vi "serverSide.vi"(1 "file path (use dialog)":path, 2 "Cluster":cluster{"Time Stamp":timestamp, "Numeric":i32}) -> ()   [LabVIEW 2017]
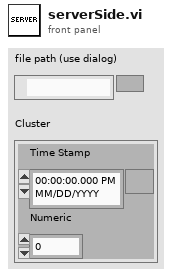
[diagram p1: front panel]
types:
  T1 = enum16{"open", "replace", "create", "open or create", "replace or create", "replace or create with confirmation"}
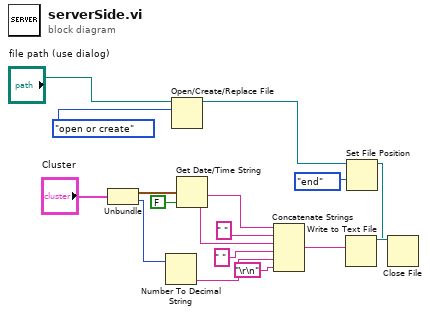
[diagram p0: block diagram]
diagram:
  n1 = Unbundle("Cluster") -> ("Time Stamp"=w2:timestamp, "Numeric"=w14:i32)
  n2 = Number To Decimal String(number=w14) -> (decimal integer string=w16:string)  [unwired: 1 in]
  n3 = Open/Create/Replace File(file path (use dialog)="file path (use dialog)", operation (0:open)=T1."open or create") -> (refnum out=w11:refnum<file>)  [unwired: 4 in, 2 out]
  n4 = Get Date/Time String(seconds (now)=w2, want seconds? (F)=FALSE) -> (date string=w3:string, time string=w5:string)  [unwired: 1 in]
  n5 = Concatenate Strings(w3, " " ("string"), w5, " " ("string"), w16, "\r\n") -> (w6:string)
  n6 = Set File Position(refnum=w11, from (0:start)=enum16{"start", "end", "current"}."end") -> (refnum out=w8:refnum<file>)  [unwired: 2 in, 1 out]
  n7 = Write to Text File(file (use dialog)=w8, text=w6) -> (refnum out=w12:refnum<file>)  [unwired: 2 in, 2 out]
  n8 = Close File(refnum=w12) -> ()  [unwired: 1 in, 2 out]
